vi "Save PID to File.vi"(8 "error in":errorcluster, 9 "PID":T1, 10 "Name":string, 11 "refnum in":T2) -> (0 "error out":errorcluster, 3 "refnum out":T2)   [LabVIEW 2016]
uses:
  <vilib>/Utility/config.llb/Config Data RefNum.ctl
  PID Settings.ctl
  <vilib>/Utility/config.llb/Write Key (Double).vi
  <vilib>/Utility/config.llb/NI_LVConfig.lvlib
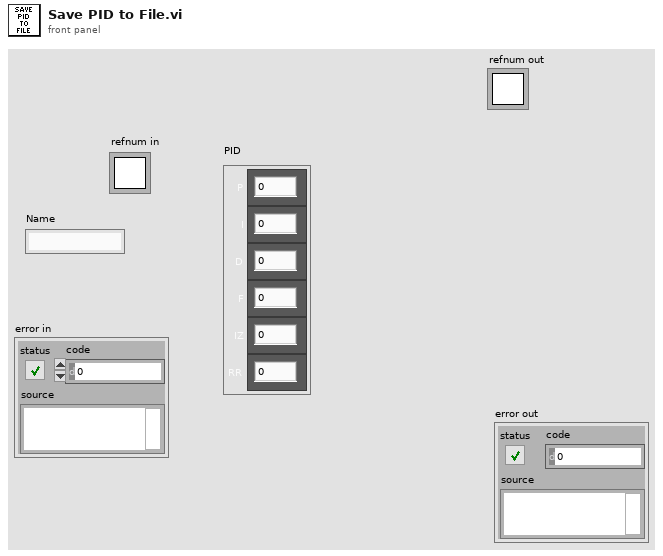
[diagram p1: front panel]
types:
  T1 = typedef "PID Settings.ctl" = cluster{"D":dbl, "F":dbl, "RR":dbl, "IZ":dbl, "P":dbl, "I":dbl}
  T2 = typedef "NI_LVConfig.lvlib/Config Data RefNum.ctl" = refnum<k1>
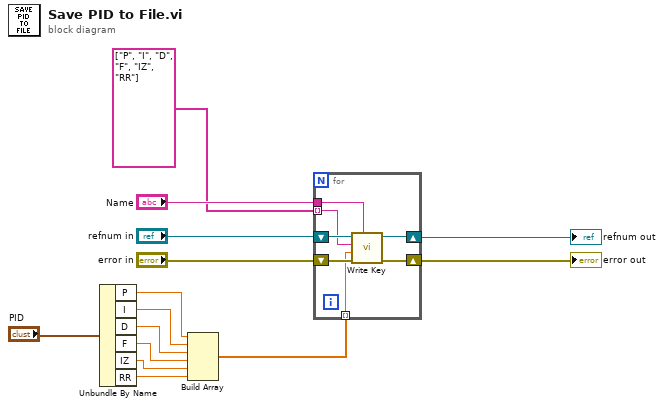
[diagram p0: block diagram]
diagram:
  n1 = Unbundle By Name("PID") -> ("P"=w7:dbl, "I"=w6:dbl, "D"=w5:dbl, "F"=w4:dbl, "IZ"=w3:dbl, "RR"=w2:dbl)
  n2 = Build Array(w7, w6, w5, w4, w3, w2) -> (w1:dbl[])
  n3 = for {
    tunnel: "Name" -> [w17]
    tunnel: string[] ["P", "I", "D", "F", "IZ", "RR"] -> [w18] mode=indexing
    shift-right: [w19] -> w9
    shift-left: "error in" -> [w20]
    shift-right: [w16] -> w10
    shift-left: "refnum in" -> [w21]
    tunnel: w1 -> [w15] mode=indexing
    n4 = call-poly <vilib>:"Write Key.vi"("section"=w17, "error in (no error)"=w20, "value"=w15, "key"=w18, "refnum"=w21) -> ("error out"=w19:errorcluster, "refnum out"=w16:T2)  [unwired: 4 in, 1 out]
  }
  "refnum out" <- w10
  "error out" <- w9
